vi "Convert String to number.vi"(1 "String":string) -> (0 "x+y":dbl)   [LabVIEW 2024]
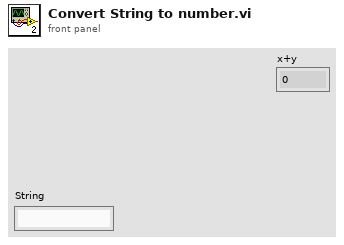
[diagram p1: front panel]
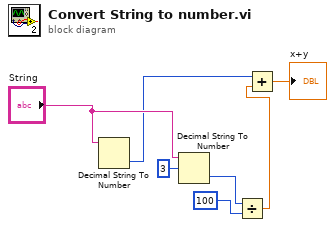
[diagram p0: block diagram]
diagram:
  n1 = Decimal String To Number(string="String") -> (number=w3:i32)  [unwired: 2 in, 1 out]
  n2 = Decimal String To Number(string="String", offset=3) -> (number=w5:i32)  [unwired: 1 in, 1 out]
  n3 = Divide(x=w5, y=100) -> (x/y=w4:dbl)
  n4 = Add(x=w3, y=w4) -> (x+y=→"x+y":dbl)
